vi "BubbleMove.vi"(8 "error in (no error)":errorcluster, 9 "Destination Index":i32, 10 "Current Index":i32, 11 "BufferedArray in":refnum<class "BufferedArray.lvclass">) -> (0 "error out":errorcluster, 3 "BufferedArray out":refnum<class "BufferedArray.lvclass">)   [LabVIEW 2013, in "LapDog.Collections.v1.Lists.Implementations.lvlib" / "BufferedArray.lvclass"]
doc: "Moves an array element from Current Index to Destination Index while maintaining the order of all the remaining elements. Current Index identfies the element to move. Destination Index is the position in the array where the element should be located.\n\nBehavior is undefined if Current Index or Destination Index is beyond the array bounds."
uses:
  BufferedArray.lvclass
  BufferedArray.lvclass/BufferedArray.ctl
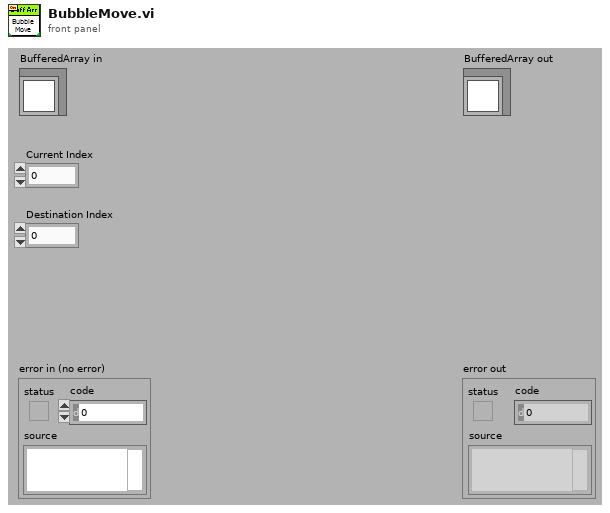
[diagram p1: front panel]
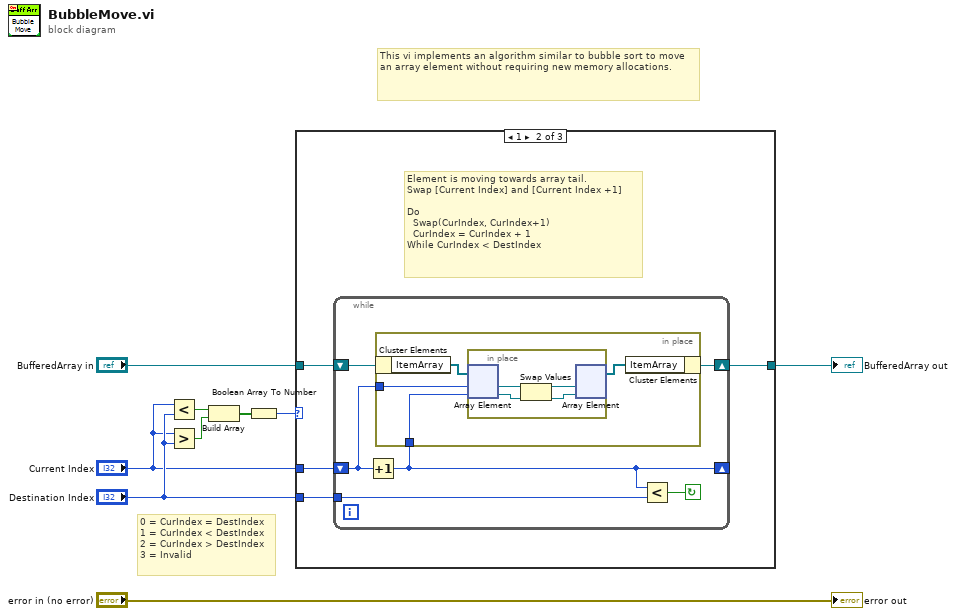
[diagram p0: block diagram]
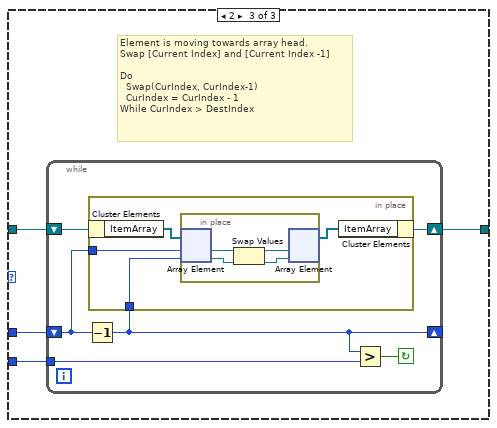
[diagram p3: hidden frame]
diagram:
  # "This vi implements an algorithm similar to bubble sort to move an array element without requiring new memory allocations."
  # "0 = CurIndex = DestIndex\n1 = CurIndex < DestIndex\n2 = CurIndex > DestIndex\n3 = Invalid"
  n1 = Less?(x="Current Index", y="Destination Index") -> (x < y?=w4:bool)
  n2 = Greater?(x="Current Index", y="Destination Index") -> (0:w3:bool)
  n3 = Build Array(w4, w3) -> (w2:bool[])
  n4 = Boolean Array To Number(Boolean array=w2) -> (number=w1:u32)
  n5 = case shown="1" w1 {
    tunnel: "BufferedArray in" -> [w10 w14 w32]
    tunnel: [w10 w13 w31] -> w7
    tunnel: "Current Index" -> [_ w12 w30]
    tunnel: "Destination Index" -> [_ w11 w29]
    frame Default {
      # "If 0, Current Index = Desitination Index.  Do nothing.\nAll other values are invalid.  Do nothing."
    }
    frame 1 {
      # "Element is moving towards array tail.\nSwap [Current Index] and [Current Index +1]\n\nDo\n  Swap(CurIndex, CurIndex+1)\n  CurIndex = CurIndex + 1\nWhile CurIndex < DestIndex"
      n6 = while {
        shift-right: [w19] -> w13
        shift-left: w14 -> [w20]
        tunnel: w11 -> [w17]
        shift-right: [w15] -> _
        shift-left: w12 -> [w16]
        stop <- w18 continue-if-true
        n7 = Increment(x=w16) -> (x+1=w15:i32)
        n8 = in-place {
          in-place-border: w16 -> [w22]
          in-place-border: w15 -> [w21]
          n9 = in-place-cluster #1(w20) -> ("ItemArray"=w24:refnum<class>[])
          n10 = in-place {
            n11 = in-place-array #2(w24, w22, w21) -> (w28:refnum<class>, w27:refnum<class>)
            n12 = Swap Values(12:w28, 14:w27) -> (1:w26:refnum<class>, 3:w25:refnum<class>)  [unwired: 1 in]
            n13 = in-place-array #2(w26, w25) -> (w23:refnum<class>[])  [unwired: 2 out]
          }
          n14 = in-place-cluster #1("ItemArray"=w23) -> (w19:refnum<class "BufferedArray.lvclass">)
        }
        n15 = Less?(x=w15, y=w17) -> (x < y?=w18:bool)
      }
    }
    frame 2 {
      # "Element is moving towards array head.\nSwap [Current Index] and [Current Index -1]\n\nDo\n  Swap(CurIndex, CurIndex-1)\n  CurIndex = CurIndex - 1\nWhile CurIndex > DestIndex"
      n16 = while {
        shift-right: [w37] -> w31
        shift-left: w32 -> [w38]
        tunnel: w29 -> [w35]
        shift-right: [w33] -> _
        shift-left: w30 -> [w34]
        stop <- w36 continue-if-true
        n17 = Decrement(x=w34) -> (x-1=w33:i32)
        n18 = in-place {
          in-place-border: w34 -> [w40]
          in-place-border: w33 -> [w39]
          n19 = in-place-cluster #3(w38) -> ("ItemArray"=w42:refnum<class>[])
          n20 = in-place {
            n21 = in-place-array #4(w42, w40, w39) -> (w46:refnum<class>, w45:refnum<class>)
            n22 = Swap Values(12:w46, 14:w45) -> (1:w44:refnum<class>, 3:w43:refnum<class>)  [unwired: 1 in]
            n23 = in-place-array #4(w44, w43) -> (w41:refnum<class>[])  [unwired: 2 out]
          }
          n24 = in-place-cluster #3("ItemArray"=w41) -> (w37:refnum<class "BufferedArray.lvclass">)
        }
        n25 = Greater?(x=w33, y=w35) -> (0:w36:bool)
      }
    }
  }
  "BufferedArray out" <- w7
  "error out" <- "error in (no error)"
